vi "VGS Automated Evaluation.vi"() -> ()   [LabVIEW 2022 SP3, in "LV_VGS.lvlib"]
uses:
  LV_VGS.lvlib
  typedefs/TaskInfo.ctl
  RemoteControlClient/VGS_RemoteControlClient.lvclass
  Job/VGS_Job.lvclass
panel:
  out "Task Info":T1
  out "getEvaluationState 1":i32(ring)=1448165568 items=["Undefined"=1448165568, "Valid"=1448165569, "OutOfTolerance"=1448165570, "InProgress"=1448165571, "NoTolerance"=1448165572]
  out "getEvaluationState 2":i32(ring)=1448165568 items=["Undefined"=1448165568, "Valid"=1448165569, "OutOfTolerance"=1448165570, "InProgress"=1448165571, "NoTolerance"=1448165572]
  # "Original evaluation Example rewritten in LabVIEW"
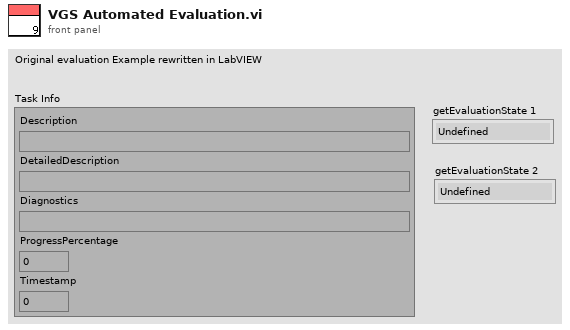
[diagram p1: front panel]
types:
  T1 = typedef "LV_VGS.lvlib/TaskInfo.ctl" = cluster{"Description":string, "DetailedDescription":string, "Diagnostics":string, "ProgressPercentage":sgl, "Timestamp":dbl}
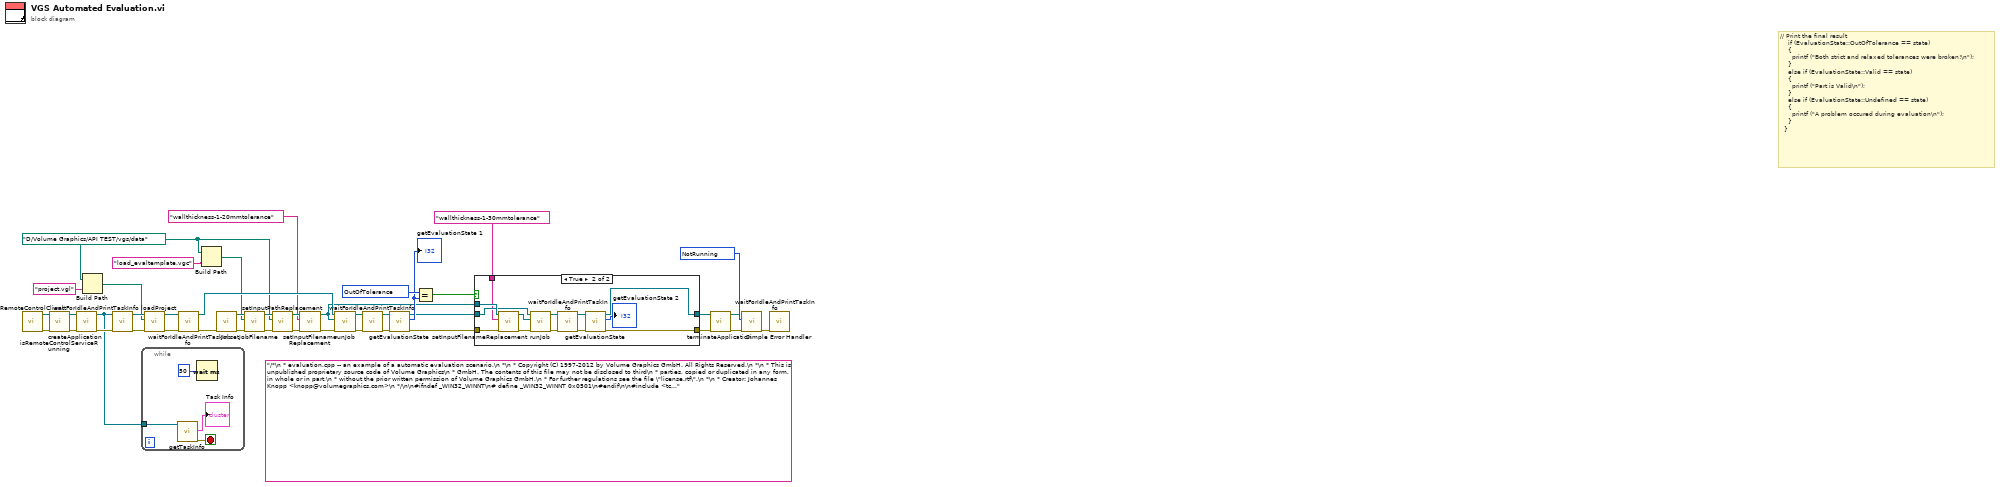
[diagram p0: block diagram]
diagram:
  (unwired) "/*\n * evaluation.cpp -- an example of a automatic evaluation scenario.\n *\n * Copyright (C) 1997-2012 by Volume Graphics GmbH. All Rights Reserved.\n *\n * This is unpublished proprietary source code of Volume Graphics\n * GmbH. The contents of this file may not be disclosed to third\n * parties, copied or duplicated in any form, in whole or in part,\n * without the prior written permission of Volume Graphics GmbH.\n * For further regulations see the file \"license.rtf\".\n *\n * Creator: Johannes Knopp <knopp@volumegraphics.com>\n */\n\n#ifndef _WIN32_WINNT\n# define _WIN32_WINNT 0x0501\n#endif\n\n#include <tchar.h>\n#include <windows.h>\n\n#include <vgs.project/error.h>\n#include <vgs.project/remotecontrolclient.h>\n\nusing namespace vgs::project;\nusing namespace vgs::project::remotecontrol;\n\nnamespace settings\n{\n  //============================== ADAPT THESE SETTINGS TO YOUR SYSTEM ========================================\n  std::string const Localhost                  (\"127.0.0.1\");                        // change this if you do not run the RCS/VGStudio (Max) on the same machine as this sample\n  int const         ServicePort = 9002;                                              // standard port, change if you chose a different port during RCS installation\n\n  //std::string const SDKDataDirectory           (\"c:\\\\sdk\\\\data\");                    // change this to the directory containing the data files delievered with the sdk\n  std::string const SDKDataDirectory           (\"D:\\\\Volume Graphics\\\\API TEST\\\\vgs\\\\data\");\n  std::string const ProjectFilename            (\"project.vgl\");                      // sample project, contained in /data folder of the sdk package\n  std::string const MacroFilename              (\"load_evaltemplate.vgc\");            // creates a surface determination and load an evaluation template, contained in /data folder\n  std::string const EvalTemplateFileBasenameA  (\"wallthickness-1-20mmtolerance\");    // sample evaluation template, contained in /data folder - use only the base name here!\n  std::string const EvalTemplateFileBasenameB  (\"wallthickness-1-30mmtolerance\");    // another sample evaluation template, contained in /data folder - use only the base name here!\n  std::string const Separator                  (\"\\\\\");\n}\n\nstatic RemoteHandle* sHandle = NULL;\n\n/*! \n  This class, once instanciated, will register itself with the global error handler.\n  It will print any occuring error messages. Should the error be that our global remote \n  handle sHandle is no longer valid, it will set it to NULL.\n*/\nclass MyErrorCallback : public Error::Callback \n{\npublic:\n  MyErrorCallback () :\n    Error::Callback ()\n  {\n    Error::setErrorCallback (this);\n  }\n\n  bool callback (const Error::ErrorCode& message)\n  {\n    if (message == Error::InvalidRemoteHandle)\n    {\n      // lost connection to VGStudio (MAX)\n      printf (\"Lost connection to current VGStudio(MAX) instance.\\n\");\n      sHandle = NULL;\n    }\n    else\n    {\n      printf (Error::getErrorDescription (message).c_str ());\n    }\n    return true;\n  }\n};\n\nvoid waitForIdleAndPrintTaskInfo (RemoteControlClient& client)\n{\n  ApplicationState::Enum appState;\n  TaskInfo info;\n  do\n  {\n    printf (Error::getErrorDescription (Error::getLastError ()).c_str ());\n    client.getTaskInfo (sHandle, info);\n    printf (\"Task: %s - %f - Diag: %s\\n\", info.Description.c_str (), info.ProgressPercentage,\n            info.Diagnostics.c_str ());\n\n    Sleep (500);\n\n    if (sHandle == NULL)\n    {\n      break;\n    }\n    client.getApplicationState (sHandle, appState);\n  }\n  while (appState != ApplicationState::Idle);\n}\n\nint _tmain (int argc, _TCHAR* argv[])\n{\n  RemoteHandle* handle = NULL;\n\n  MyErrorCallback     callback;                           // Create an instance of MyErrorCallback.  \n  RemoteControlClient client (settings::Localhost, settings::ServicePort);  // Create a client for communication with the target system\n\n  // Check if the service is available on the target system\n  {\n    if (true != client.isRemoteControlServiceRunning ())\n    {\n      printf (\"Service isn't available on %s:%d.\\n\", settings::Localhost, settings::ServicePort);\n      return -1;\n    }\n  }\n\n  ApplicationState::Enum appState;\n\n  // Start a VGStudio (MAX) instance\n  printf (\"Starting VGStudio (MAX) \");\n  {\n    sHandle = client.createApplication (ApplicationVisibility::Visible);\n    if (NULL == sHandle)\n    {\n      printf (\"Unable to create VGStudio (MAX) instance.\\n\");\n      Error::ErrorCode err = Error::getLastError ();\n      __debugbreak ();\n      return -1;\n    }\n\n    // Wait until the application is in an idle state\n    do\n    {\n      printf (\".\");\n      if (sHandle == NULL)\n      {\n        break;\n      }\n      client.getApplicationState (sHandle, appState);\n\n      Sleep (500);  // Wait half a second until we poll the state again\n    }\n    while (appState != ApplicationState::Idle);\n  }\n  printf (\"\\n\");\n\n  Sleep (1000); // wait a second\n\n  // Load a project containing the volume that we want to evaluate.\n  {\n    if (true != client.loadProject (sHandle, settings::SDKDataDirectory + settings::Separator + settings::ProjectFilename))\n    {\n      Error::ErrorCode err = Error::getLastError ();\n      __debugbreak ();\n      return -1;\n    }\n\n    waitForIdleAndPrintTaskInfo (client);\n  }\n\n  if (Error::getLastError () != Error::NoError)\n  {\n    Error::ErrorCode err = Error::getLastError ();\n    __debugbreak ();\n    return -1;\n  }\n\n  // Create a Job that will execute a macro, which in turn will load an evaluation template.\n  // The sample evaluation template will create a wallthickness analysis and evaluate its' result.\n  Job evaluationJob;\n  evaluationJob.setJobFilename  (settings::SDKDataDirectory + settings::Separator + settings::MacroFilename);  // set the path to the macro\n\n  // The macro stores the path to the template as it was when the macro was recorded. Since\n  // the position of this template on disk may have changed since then, we have to make sure\n  // the macro can find it again. This is done via a replacement object that we attach to the\n  // job object.\n  // This way, we can use the same macro to play back different evaluation templates.\n  Job::FilenameReplacement filenameReplacement  (settings::EvalTemplateFileBasenameA); // new filename is one of the sample evaluation templates\n  Job::PathReplacement     pathReplacement      (settings::SDKDataDirectory);          // new path is the working directory\n\n  evaluationJob.setInputPathReplacement     (pathReplacement);                // attach new path to the job\n  evaluationJob.setInputFilenameReplacement (filenameReplacement);            // attach new filename to the job\n\n  // Now that the project has been loaded and the job prepared, we run it.\n  {\n    if (true != client.runJob (sHandle, evaluationJob))\n    {\n      Error::ErrorCode err = Error::getLastError ();\n      __debugbreak ();\n      return -1;\n    }\n\n    waitForIdleAndPrintTaskInfo (client);\n  }\n\n  if (Error::getLastError () != Error::NoError)\n  {\n    Error::ErrorCode err = Error::getLastError ();\n    __debugbreak ();\n    return -1;\n  }\n\n  // The macro has been successfully played back - now we can query the result of the evaluation\n  // loaded via the evaluation template.\n  EvaluationState::Enum state;      // this will store the state of our evaluation\n\n  {\n    if (true != client.getEvaluationState (sHandle, state))\n    {\n      Error::ErrorCode err = Error::getLastError ();\n      __debugbreak ();\n      return -1;\n    }\n  }\n\n  // Depending on the state of the evaluation, we react in a certain way.\n  // In case the tolerance was broken, we try an evaluation template containing a less strict tolerance.\n  bool tryLessStrict = false;\n\n  if (EvaluationState::OutOfTolerance == state)\n  {\n    printf (\"Part is OutOfTolerance. Trying relaxed tolerance!\\n\");\n    tryLessStrict = true;\n  }\n  else if (EvaluationState::Valid == state)\n  {\n    printf (\"Part is Valid\\n\");\n  }\n  else if (EvaluationState::Undefined == state)\n  {\n    printf (\"A problem occured during evaluation\\n\");\n  }\n\n  if (tryLessStrict)\n  {\n    Job::FilenameReplacement lessStrictTemplate (settings::EvalTemplateFileBasenameB);\n    evaluationJob.setInputFilenameReplacement (lessStrictTemplate);\n\n    // Run the modified job with the less strict template.\n    {\n      if (true != client.runJob (sHandle, evaluationJob))\n      {\n        Error::ErrorCode err = Error::getLastError ();\n        __debugbreak ();\n        return -1;\n      }\n\n      waitForIdleAndPrintTaskInfo (client);\n    }\n\n    // Query the evaluation state again\n    {\n      if (true != client.getEvaluationState (sHandle, state))\n      {\n        Error::ErrorCode err = Error::getLastError ();\n        __debugbreak ();\n        return -1;\n      }\n    }\n  \n    // Print the final result\n    if (EvaluationState::OutOfTolerance == state)\n    {\n      printf (\"Both strict and relaxed tolerances were broken!\\n\");\n    }\n    else if (EvaluationState::Valid == state)\n    {\n      printf (\"Part is Valid\\n\");\n    }\n    else if (EvaluationState::Undefined == state)\n    {\n      printf (\"A problem occured during evaluation\\n\");\n    }\n  }\n\n  // stop VGStudio (MAX)\n  {\n    if (true != client.terminateApplication (sHandle))\n    {\n      Error::ErrorCode err = Error::getLastError ();\n      __debugbreak ();\n\n      return -1;\n    }\n\n    // wait for finish\n    printf (\"Stopping VGStudio (MAX) \");\n    do\n    {\n      Sleep (500);\n      printf (\".\");\n\n      if (sHandle == NULL)\n      {\n        break;\n      }\n      client.getApplicationState (sHandle, appState);\n    }\n    while (appState != ApplicationState::NotRunning);\n    printf (\"\\n\");\n\n    printf (\"Done.\\n\");\n    sHandle = NULL;\n  }\n\n  getchar ();\n\n  return 0;\n}\n\n"
  w4 = path "D:/Volume Graphics/API TEST/vgs/data" ("replacementPattern")
  w11 = 1448165376 items=["NotRunning"=1448165376, "Starting"=1448165377, "Dying"=1448165378, "Idle"=1448165379, "WorkInProgress"=1448165380] ("wait for ApplicationState (Idle)")
  w20 = 1448165570 items=["Undefined"=1448165568, "Valid"=1448165569, "OutOfTolerance"=1448165570, "InProgress"=1448165571, "NoTolerance"=1448165572] ("getEvaluationState")
  # "// Print the final result\n    if (EvaluationState::OutOfTolerance == state)\n    {\n      printf (\"Both strict and relaxed tolerances were broken!\\n\");\n    }\n    else if (EvaluationState::Valid == state)\n    {\n      printf (\"Part is Valid\\n\");\n    }\n    else if (EvaluationState::Undefined == state)\n    {\n      printf (\"A problem occured during evaluation\\n\");\n    }\n  }"
  n1 = call "RemoteControlClient.vi"() -> ("error out"=w41:errorcluster, "VGS_RemoteControlClient out"=w42:refnum<class "VGS_RemoteControlClient.lvclass">)  [unwired: 10 in]
  n2 = call "isRemoteControlServiceRunning.vi"("error in (no error)"=w41, "VGS_RemoteControlClient in"=w42) -> ("error out"=w40:errorcluster, "VGS_RemoteControlClient out"=w39:refnum<class "VGS_RemoteControlClient.lvclass">)  [unwired: 7 in, 1 out]
  n3 = call "createApplication.vi"("error in (no error)"=w40, "VGS_RemoteControlClient in"=w39) -> ("error out"=w38:errorcluster, "VGS_RemoteControlClient out"=w7:refnum<class "VGS_RemoteControlClient.lvclass">)  [unwired: 8 in]
  n4 = Build Path(base path=w4, name or relative path="project.vgl") -> (appended path=w2:path)
  n5 = call "waitForIdleAndPrintTaskInfo.vi"("error in (no error)"=w38, "VGS_RemoteControlClient in"=w7) -> ("error out"=w37:errorcluster, "VGS_RemoteControlClient out"=w36:refnum<class "VGS_RemoteControlClient.lvclass">)  [unwired: 8 in]
  n6 = while {
    tunnel: w7 -> [w45]
    stop <- w44 stop-if-true
    n7 = call "getTaskInfo.vi"("VGS_RemoteControlClient in"=w45) -> ("error out"=w44:errorcluster, "Task Info"=→"Task Info":T1)  [unwired: 7 in, 2 out]
    n8 = Wait (ms)(milliseconds to wait=u32 50) -> ()  [unwired: 1 out]
  }
  n9 = call "loadProject.vi"("error in (no error)"=w37, "projectName"=w2, "VGS_RemoteControlClient in"=w36) -> ("error out"=w35:errorcluster, "VGS_RemoteControlClient out"=w34:refnum<class "VGS_RemoteControlClient.lvclass">)  [unwired: 7 in]
  n10 = call "waitForIdleAndPrintTaskInfo.vi"("error in (no error)"=w35, "VGS_RemoteControlClient in"=w34) -> ("error out"=w27:errorcluster, "VGS_RemoteControlClient out"=w25:refnum<class "VGS_RemoteControlClient.lvclass">)  [unwired: 8 in]
  n11 = Build Path(base path=w4, name or relative path="load_evaltemplate.vgc") -> (appended path=w5:path)
  n12 = call "Job.vi"("error in (no error)"=w27) -> ("error out"=w32:errorcluster, "VGS_Job out"=w33:refnum<class "VGS_Job.lvclass">)  [unwired: 9 in]
  n13 = call "setJobFilename.vi"("error in (no error)"=w32, "Path to Job File"=w5, "VGS_Job in"=w33) -> ("error out"=w29:errorcluster, "VGS_Job out"=w31:refnum<class "VGS_Job.lvclass">)  [unwired: 7 in]
  n14 = call "setInputPathReplacement.vi"("error in (no error)"=w29, "replacementPattern"=w4, "VGS_Job in"=w31) -> ("error out"=w28:errorcluster, "VGS_Job out"=w30:refnum<class "VGS_Job.lvclass">)  [unwired: 7 in]
  n15 = call "setInputFilenameReplacement.vi"("error in (no error)"=w28, "replacementPattern"="wallthickness-1-20mmtolerance", "VGS_Job in"=w30) -> ("error out"=w26:errorcluster, "VGS_Job out"=w16:refnum<class "VGS_Job.lvclass">)  [unwired: 7 in]
  n16 = call "runJob.vi"("error in (no error)"=w26, "VGS_Job in"=w16, "VGS_RemoteControlClient in"=w25) -> ("error out"=w24:errorcluster, "VGS_RemoteControlClient out"=w23:refnum<class "VGS_RemoteControlClient.lvclass">)  [unwired: 7 in]
  n17 = call "waitForIdleAndPrintTaskInfo.vi"("error in (no error)"=w24, "VGS_RemoteControlClient in"=w23) -> ("error out"=w21:errorcluster, "VGS_RemoteControlClient out"=w22:refnum<class "VGS_RemoteControlClient.lvclass">)  [unwired: 8 in]
  n18 = call "getEvaluationState.vi"("error in (no error)"=w21, "VGS_RemoteControlClient in"=w22) -> ("error out"=w15:errorcluster, "getEvaluationState"=w18:i32, "VGS_RemoteControlClient out"=w17:refnum<class "VGS_RemoteControlClient.lvclass">)  [unwired: 7 in]
  "getEvaluationState 1" <- w18
  n19 = Equal?(x=w20, y=w18) -> (x = y?=w19:bool)
  n20 = case shown="True" w19 {
    tunnel: w17 -> [w47 w59]
    tunnel: w16 -> [_ w61]
    tunnel: w15 -> [w48 w60]
    tunnel: [w48 w52] -> w14
    tunnel: [w47 w51] -> w13
    tunnel: "wallthickness-1-30mmtolerance" ("replacementPattern") -> [_ w49]
    frame False {
    }
    frame True {
      n21 = call "setInputFilenameReplacement.vi"("error in (no error)"=w60, "replacementPattern"=w49, "VGS_Job in"=w61) -> ("error out"=w57:errorcluster, "VGS_Job out"=w58:refnum<class "VGS_Job.lvclass">)  [unwired: 7 in]
      n22 = call "runJob.vi"("error in (no error)"=w57, "VGS_Job in"=w58, "VGS_RemoteControlClient in"=w59) -> ("error out"=w56:errorcluster, "VGS_RemoteControlClient out"=w55:refnum<class "VGS_RemoteControlClient.lvclass">)  [unwired: 7 in]
      n23 = call "waitForIdleAndPrintTaskInfo.vi"("error in (no error)"=w56, "VGS_RemoteControlClient in"=w55) -> ("error out"=w54:errorcluster, "VGS_RemoteControlClient out"=w53:refnum<class "VGS_RemoteControlClient.lvclass">)  [unwired: 8 in]
      n24 = call "getEvaluationState.vi"("error in (no error)"=w54, "VGS_RemoteControlClient in"=w53) -> ("error out"=w52:errorcluster, "getEvaluationState"=→"getEvaluationState 2":i32, "VGS_RemoteControlClient out"=w51:refnum<class "VGS_RemoteControlClient.lvclass">)  [unwired: 7 in]
    }
  }
  n25 = call "terminateApplication.vi"("error in (no error)"=w14, "VGS_RemoteControlClient in"=w13) -> ("error out"=w12:errorcluster, "VGS_RemoteControlClient out"=w10:refnum<class "VGS_RemoteControlClient.lvclass">)  [unwired: 8 in]
  n26 = call "waitForIdleAndPrintTaskInfo.vi"("error in (no error)"=w12, "wait for ApplicationState (Idle)"=w11, "VGS_RemoteControlClient in"=w10) -> ("error out"=w9:errorcluster)  [unwired: 7 in, 1 out]
  n27 = call <vilib>:"Simple Error Handler.vi"("error in (no error)"=w9) -> ()  [unwired: 4 in, 5 out]
